vi "fgv_Chirp Paremeters other.vi"(6 "Imaging Protocol in":T1, 8 "error in":errorcluster, 9 "Function":T2, 11 "Chirps in":cluster{"HexPackets":string[]}) -> (0 "error out":errorcluster, 2 "Imaging Protocol":T1, 3 "Chirps":cluster{"HexPackets":string[]})   [LabVIEW 2013]
uses:
  Typedefs/Read Write Enum.ctl
  Typedefs/Imaging Protocols enum.ctl
panel:
  # "SUBROUTINE"
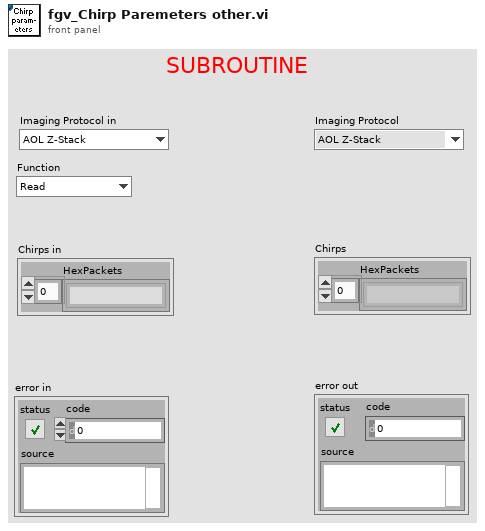
[diagram p1: front panel]
types:
  T1 = typedef "Imaging Protocols enum.ctl" = enum16{"AOL Z-Stack", "Motor Z Stack", "Functional Acquisition", "Single Plane Acquisition", "Volume Acquisition", "Live Imaging", "Live Plane Imaging", "Live Volume Imaging"}
  T2 = typedef "Read Write Enum.ctl" = enum16{"Read", "Write"}
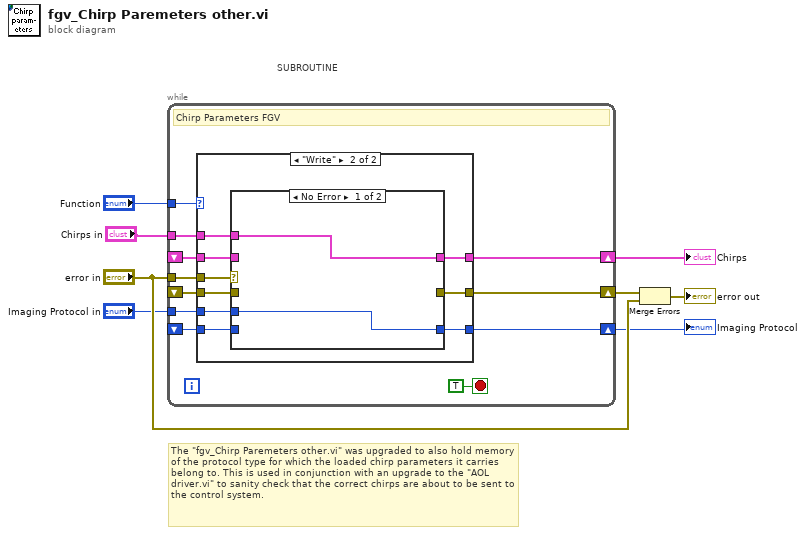
[diagram p0: block diagram]
diagram:
  # "The \"fgv_Chirp Paremeters other.vi\" was upgraded to also hold memory of the protocol type for which the loaded chirp parameters it carries belong to. This is used in conjunction with an upgrade to the \"AOL driver.vi\" to sanity check that the correct chirps are about to be sent to the control system."
  # "SUBROUTINE"
  n1 = while {
    tunnel: "Function" -> [w18]
    tunnel: "Chirps in" -> [w17]
    shift-right: [w16] -> w3
    shift-left: _ -> [w15]
    tunnel: "error in" -> [w14]
    shift-right: [w13] -> w7
    shift-left: _ -> [w12]
    tunnel: "Imaging Protocol in" -> [w11]
    shift-right: [w10] -> w1
    shift-left: _ -> [w9]
    stop <- TRUE stop-if-true
    # "Chirp Parameters FGV"
    n2 = case shown="\"Write\"" w18 {
      tunnel: w17 -> [_ w30]
      tunnel: [w22 w29] -> w16
      tunnel: w15 -> [w22 w28]
      tunnel: w14 -> [_ w31]
      tunnel: [w21 w27] -> w13
      tunnel: w12 -> [w21 w26]
      tunnel: w11 -> [_ w25]
      tunnel: [w20 w24] -> w10
      tunnel: w9 -> [w20 w23]
      frame "Read", Default {
      }
      frame "Write" {
        n3 = case shown="No Error" w31 {
          selector: w31 -> [_ w35]
          tunnel: w30 -> [w33 _]
          tunnel: [w33 w36] -> w29
          tunnel: w28 -> [_ w36]
          tunnel: [_ w35] -> w27
          tunnel: w26 -> [_ _]
          tunnel: w25 -> [w32 _]
          tunnel: [w32 w34] -> w24
          tunnel: w23 -> [_ w34]
          frame No Error {
          }
          frame Error {
          }
        }
      }
    }
  }
  "Chirps" <- w3
  "Imaging Protocol" <- w1
  n4 = Merge Errors(w7, "error in") -> (→"error out":errorcluster)
